vi "PathPlanner_PathConstraints_New.vi"(8 "MaxAngularAccRadPSecSq":dbl, 9 "MaxAngularVelRadPsEc;":dbl, 10 "MaxAccelerationMpsSq;":dbl, 11 "MaxVelocityMps;":dbl) -> (3 "PathPlannerConstraints":T1)   [LabVIEW 2019, in "PathPlanner.lvlib"]
doc: "Create a new path constraints object\n\nInputs: \n - maxVelocityMps - double - Max linear velocity (M/S)\n - maxAccelerationMpsSq - double - Max linear acceleration (M/S^2)\n - maxAngularVelocityRps - double - Max angular velocity (Rad/S)\n - maxAngularAccelerationRpsSq - double - Max angular acceleration (Rad/S^2)\n\nOutputs:\n - PathConstraint - cluster - path constraint data"
uses:
  PathPlanner.lvlib
  TypeDef/PathPlannerPathConstraints.ctl
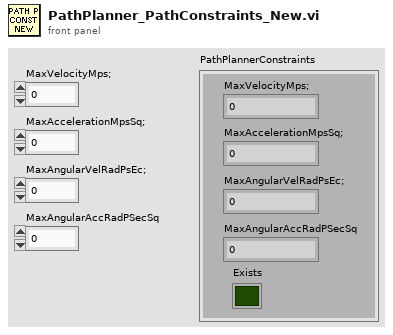
[diagram p1: front panel]
types:
  T1 = typedef "PathPlanner.lvlib/PathPlannerPathConstraints.ctl" = cluster{"MaxVelocityMps;":dbl, "MaxAccelerationMpsSq;":dbl, "MaxAngularVelRadPsEc;":dbl, "MaxAngularAccRadPSecSq":dbl, "Exists":bool}
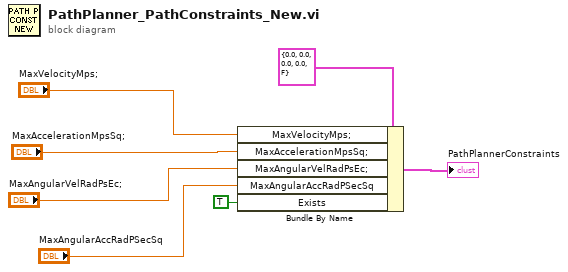
[diagram p0: block diagram]
diagram:
  n1 = Bundle By Name(cluster=T1 {"MaxVelocityMps;"=0.0, "MaxAccelerationMpsSq;"=0.0, "MaxAngularVelRadPsEc;"=0.0, "MaxAngularAccRadPSecSq"=0.0, "Exists"=FALSE} ("PathPlannerConstraints"), "MaxVelocityMps;"="MaxVelocityMps;", "MaxAccelerationMpsSq;"="MaxAccelerationMpsSq;", "MaxAngularVelRadPsEc;"="MaxAngularVelRadPsEc;", "MaxAngularAccRadPSecSq"="MaxAngularAccRadPSecSq", "Exists"=TRUE) -> (→"PathPlannerConstraints":T1)
